vi "Test particle has position.vi"(8 "error in (no error)":errorcluster, 11 "Test Case In":refnum<class "Particle Test.lvclass">) -> (0 "error out":errorcluster, 3 "Test Case Out":refnum<class "Particle Test.lvclass">)   [LabVIEW 2020, in "Particle Test.lvclass"]
uses:
  Particle Test.lvclass
  Particle Test.lvclass/Particle Test.ctl
  01074fa8-ee8a-411d-bc8b-fc92c4f90959.vi
  source/Particle.lvclass
  source/Particle/Position.ctl
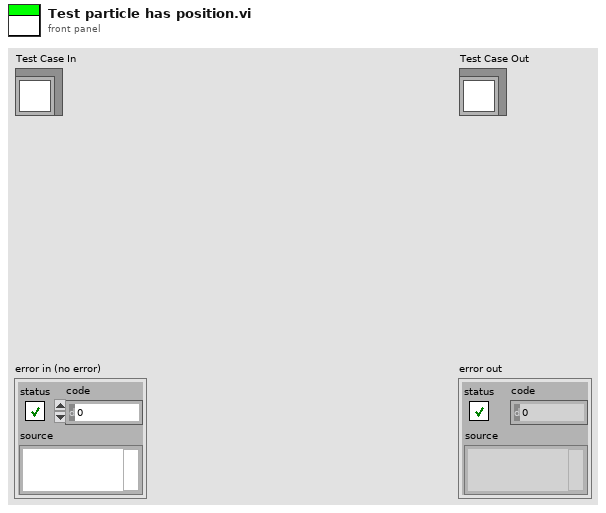
[diagram p1: front panel]
types:
  T1 = typedef "Particle.lvclass/Position.ctl" = cluster{"X":i32, "Y":i32}
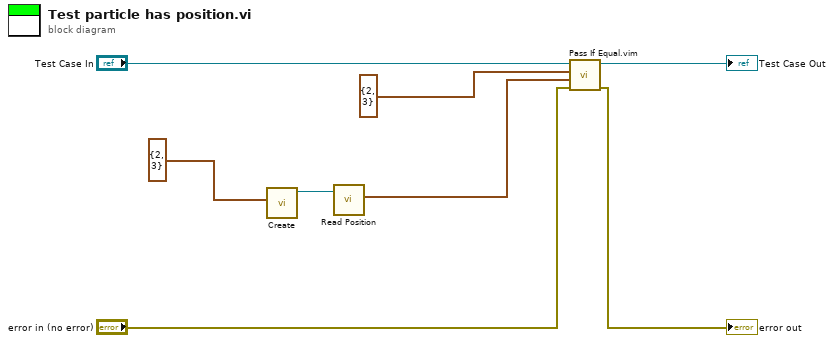
[diagram p0: block diagram]
diagram:
  n1 = call "Create.vi"("Position"=T1 {"X"=2, "Y"=3}) -> ("Particle out"=w2:refnum<class "Particle.lvclass">)  [unwired: 10 in]
  n2 = call "Read Position.vi"("Particle in"=w2) -> ("Position"=w1:T1)  [unwired: 9 in, 1 out]
  n3 = call "Pass If Equal.vim"("error in (no error)"="error in (no error)", "Actual"=w1, "Expected"=T1 {"X"=2, "Y"=3} ("Position"), "LUnit Test Case In"="Test Case In") -> ("error out"=→"error out":errorcluster, "LUnit Test Case Out"=→"Test Case Out":refnum<class "Particle Test.lvclass">)  [unwired: 6 in]
